vi "ExpBind.vi"(8 "Binding Type":T1=enum."Bidrectional", 9 "Parameter Name (use value name)":string, 10 "Value":variant, 11 "ExpID":string) -> (1 "Processed As Controls Array":bool, 3 "ExpID out":string)   [LabVIEW 2017]
uses:
  Expose/Labview/Parameters/ExposeParameterBindingType.ctl
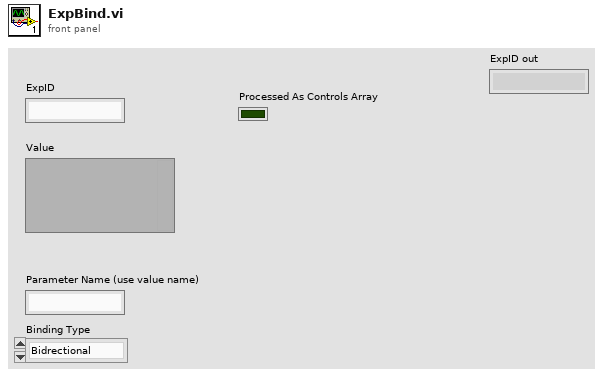
[diagram p1: front panel]
types:
  T1 = typedef "ExposeParameterBindingType.ctl" = enum16{"ToRemote", "FromRemote", "Bidrectional"}
  T2 = typedef "ExperimentInfo.ctl" = cluster{"ExposeInfo":T3, "ExpID":string, "ExperimentFilename":string, "Caller Keep Alive":refnum<data-value>}
  T3 = typedef "ExposeInfo.ctl" = cluster{"CSCom":refnum<k24>, "URL":string, "Events Category":string, "ID":string, "SRefID":string}
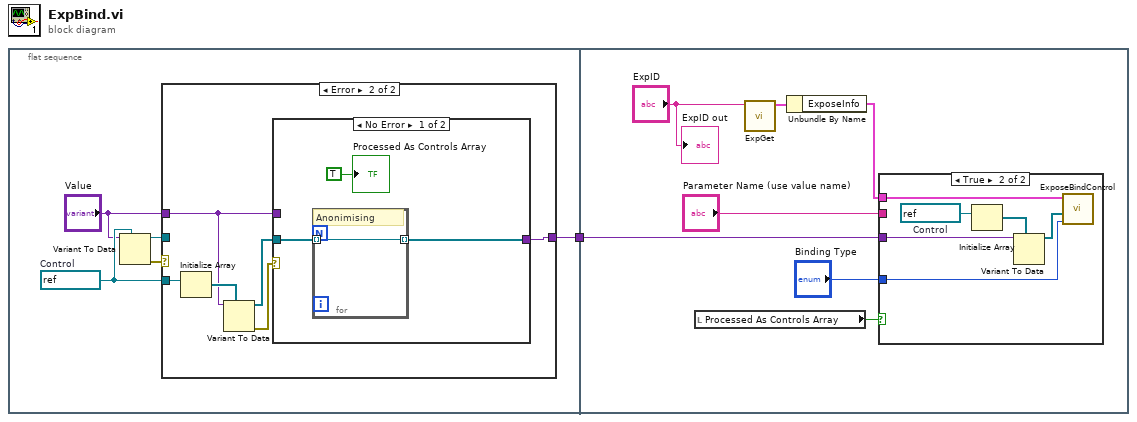
[diagram p0: block diagram]
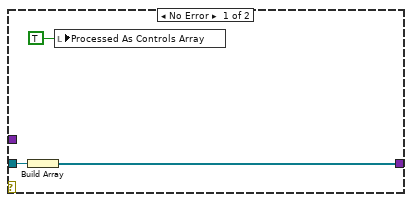
[diagram p2: hidden frame]
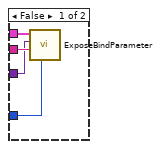
[diagram p4: hidden frame]
diagram:
  n1 = flat-sequence {
    tunnel: [w3] -> w1
    tunnel: w1 -> [w22]
    frame #0 {
      w4 = refnum<vi> refnum  # Control
      n2 = Variant To Data(type=w4, Variant="Value") -> (data=w5:refnum<vi>, error out=w6:errorcluster)  [unwired: 1 in]
      n3 = case shown="Error" w6 {
        tunnel: w5 -> [w9 _]
        tunnel: w4 -> [_ w15]
        tunnel: "Value" -> [_ w10]
        tunnel: [w8 w11] -> w3
        frame No Error {
          n4 = Build Array(w9) -> (w8:refnum<vi>[])
          n5 = local write "Processed As Controls Array"(TRUE ("Processed As Control Collection")) -> ()
        }
        frame Error {
          n6 = Initialize Array(w15) -> (w14:refnum<vi>[])  [unwired: 1 in]
          n7 = Variant To Data(type=w14, Variant=w10) -> (data=w12:refnum<vi>[], error out=w13:errorcluster)  [unwired: 1 in]
          n8 = case shown="No Error" w13 {
            tunnel: w12 -> [w17 _]
            tunnel: [w16 w20] -> w11
            tunnel: w10 -> [_ w20]
            frame No Error {
              n9 = for {
                tunnel: w17 -> [w19] mode=indexing
                tunnel: [w19] -> w16 mode=indexing
                # "Anonimising"
              }
              "Processed As Controls Array" <- TRUE ("Processed As Control Collection")
            }
            frame Error {
            }
          }
        }
      }
    }
    frame #1 {
      n10 = local read "Processed As Controls Array"() -> (w21:bool)
      n11 = call "ExpGet.vi"("ExpID"="ExpID") -> ("Exp Info"=w24:T2)  [unwired: 9 in, 1 out]
      n12 = Unbundle By Name(w24) -> ("ExposeInfo"=w25:T3)
      n13 = case shown="True" w21 {
        tunnel: w25 -> [w31 w37]
        tunnel: "Parameter Name (use value name)" -> [w30 _]
        tunnel: "Binding Type" -> [w29 w36]
        tunnel: w22 -> [w28 w35]
        frame False {
          n14 = call "ExposeBindParameter.vi"("Bind Direction"=w29, "Name (empty)"=w30, "Value"=w28, "Expose Info"=w31) -> ()  [unwired: 8 in]
        }
        frame True {
          w34 = refnum<vi> refnum  # Control
          n15 = Initialize Array(w34) -> (w33:refnum<vi>[])  [unwired: 1 in]
          n16 = Variant To Data(type=w33, Variant=w35) -> (data=w32:refnum<vi>[])  [unwired: 1 in, 1 out]
          n17 = call "ExposeBindControl.vi"("Binding Type"=w36, "Controls"=w32, "Expose Info"=w37) -> ()  [unwired: 9 in]
        }
      }
      "ExpID out" <- "ExpID"
    }
  }
